vi "Send Data to Host.vi"(8 "error in":errorcluster, 11 "PAS in":refnum<class "cPAS.lvclass">) -> (0 "error out":errorcluster, 3 "PAS out":refnum<class "cPAS.lvclass">)   [LabVIEW 2015, in "cPAS.lvclass"]
doc: "Override this VI to use it to send implementation specific commands for communicating with a host or user interface."
uses:
  cPAS.lvclass
  Reusable/PAS/Main/Read Data.vi
  Reusable/PAS/Data/Main/PAS Data.lvclass
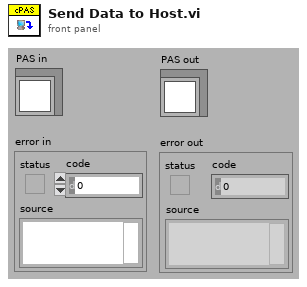
[diagram p1: front panel]
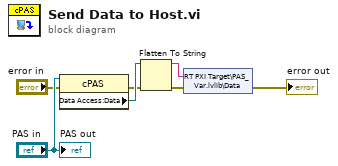
[diagram p0: block diagram]
diagram:
  n1 = property class="cPAS"(reference="PAS in", error in="error in") -> (error out=w1:errorcluster, "Data Access:Data"=w3:refnum<class "PAS Data.lvclass">)  [unwired: 1 out]
  n2 = Flatten To String(anything=w3, error in (no error)=w1) -> (data string=w7:string, error out=w6:errorcluster)  [unwired: 2 in, 1 out]
  n3 = shared-variable "RT PXI Target\\PAS_Var.lvlib\\Data"(w7, error in=w6) -> (error out=→"error out":errorcluster)
  "PAS out" <- "PAS in"
